vi "CAN Decode List File.vi"(9 "IgnoreIDListLen":i32, 10 "pIgnoreIDList":u32[](array[numeric])=[0, 0, 0, 0, 0, 0, 0, 0, 0, 0, 0, 0, 0, 0, 0, 0], 11 "pFileName":string) -> (1 "function return":i32, 2 "pIgnoreIDList out":u32[](array[numeric]), 3 "pFileName out":string)   [LabVIEW 2010, in "usb2can.lvlib"]
doc: "int WINAPI CAN_DecodeListFile(char *pFileName,unsigned int *pIgnoreIDList,int IgnoreIDListLen);"
uses:
  usb2can.lvlib
  USB2XXX.dll
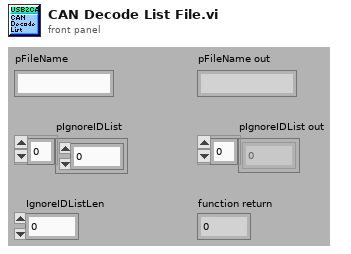
[diagram p1: front panel]
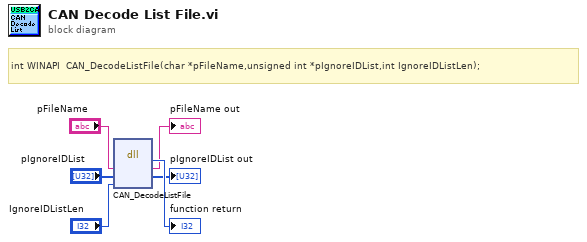
[diagram p0: block diagram]
diagram:
  # "int WINAPI  CAN_DecodeListFile(char *pFileName,unsigned int *pIgnoreIDList,int IgnoreIDListLen);"
  n1 = dll-call lib="E:/OtherWork/STM32/USB2XXX_Example/sdk/api/Labview/USB2XXX.*" fn="CAN_DecodeListFile"("pFileName"="pFileName", "pIgnoreIDList"="pIgnoreIDList", "IgnoreIDListLen"="IgnoreIDListLen") -> (→"function return":i32, "pFileName"=→"pFileName out":string, "pIgnoreIDList"=→"pIgnoreIDList out":u32[])  [unwired: 4 in, 2 out]
